vi "RTM CreateFramesChannels.vi"(8 "error in (no error)":errorcluster, 10 "Frame":string="Tx FRAME ", 11 "Node Ptr":T1 format="%.0x") -> (0 "error out":errorcluster, 3 "Node Ptr 2":T1 format="%.0x")   [LabVIEW 2018, in "CAN Gateway System Explorer.lvlib"]
uses:
  CAN Gateway System Explorer.lvlib
  <vilib>/NI Veristand/Custom Device API/Custom Device Item Ref.ctl
  <vilib>/NI Veristand/Custom Device Tools/Custom Device Utility Library/Search Direction.ctl
  <vilib>/NI Veristand/Custom Device API/Custom Device Channel.ctl
  <vilib>/NI Veristand/Custom Device API/Custom Device Channel Type.ctl
  Shared/Constants.vi
  <vilib>/NI Veristand/Custom Device Tools/Custom Device Utility Library/NI VeriStand - Search for Item by GUID.vi
  <vilib>/NI Veristand/Custom Device API/Get Item Property (String).vi
  <vilib>/NI Veristand/Custom Device API/Set Item Property (Boolean).vi
  <resource>/objmgr/xnet.rc
  <vilib>/NI Veristand/Custom Device Tools/Custom Device Utility Library/Custom Device Utility Library.lvlib
  Shared/CAN Gateway Shared.lvlib
  <vilib>/NI Veristand/Custom Device API/Custom Device API.lvlib
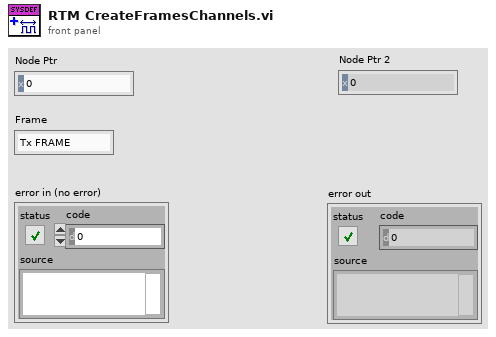
[diagram p1: front panel]
types:
  T1 = typedef "Custom Device API.lvlib/Custom Device Item Ref.ctl" = u64
  T2 = typedef "Custom Device Utility Library.lvlib/Search Direction.ctl" = enum16{"Down", "Up"}
  T3 = typedef "Custom Device API.lvlib/Custom Device Channel.ctl" = cluster{"Type":T4, "Units":string, "Default Value":dbl, "Faultable":bool, "Scalable":bool}
  T4 = typedef "Custom Device API.lvlib/Custom Device Channel Type.ctl" = enum16{"Input", "Output"}
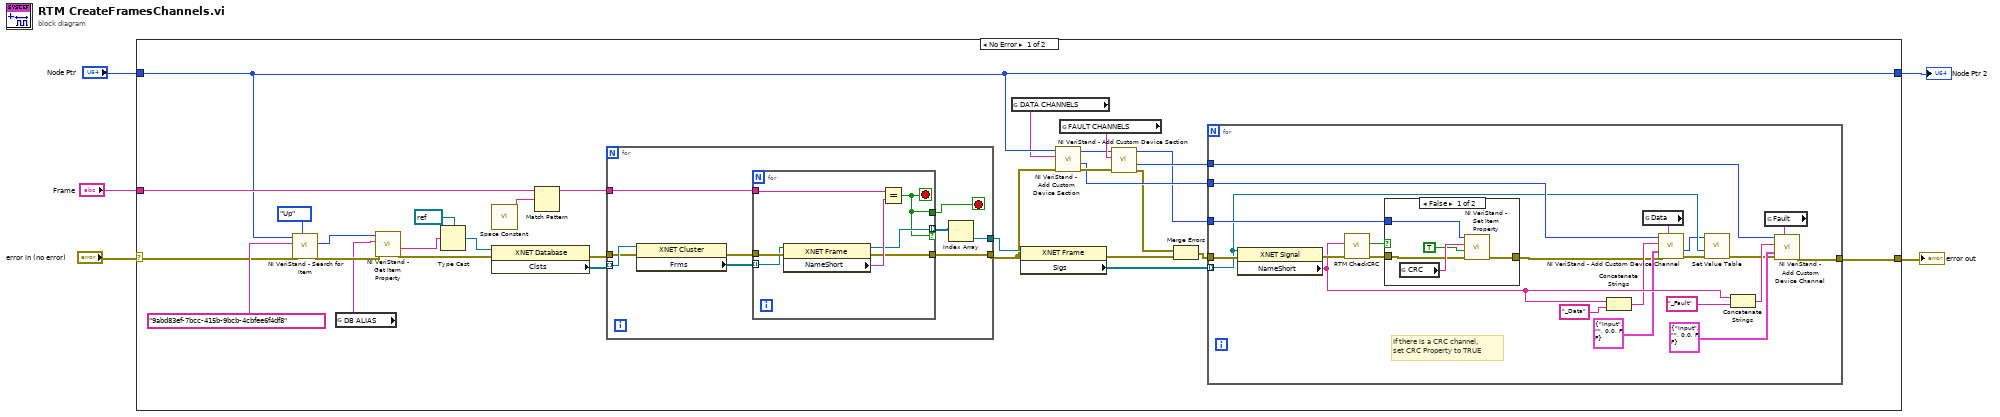
[diagram p0: block diagram]
diagram:
  n1 = case shown="No Error" "error in (no error)" {
    selector: "error in (no error)" -> [w31 w80]
    tunnel: "Node Ptr" -> [w16 w81]
    tunnel: "Frame" -> [w22 _]
    tunnel: [w16 w81] -> w2
    tunnel: [w18 w80] -> w1
    frame No Error {
      n2 = call-poly <vilib>:"NI VeriStand - Search for Item.vi"("Direction (Down)"=Search_Direction."Up", "error in"=w31, "Item GUID"="9abd83ef-7bcc-415b-9bcb-4cbfee6f4df8", "Section Ref in"=w16) -> ("error out"=w34:errorcluster, "Item Ref"=w32:T1)  [unwired: 4 in, 2 out]
      n3 = global read "Constants.vi" "DB ALIAS"() -> (w33:string)
      n4 = call-poly <vilib>:"NI VeriStand - Get Item Property.vi"("error in (no error)"=w34, "Property Name"=w33, "Item Ref in"=w32) -> ("error out"=w28:errorcluster, "Value"=w29:string)  [unwired: 5 in, 2 out]
      n5 = Type Cast(type=refnum<k21> refnum ("XNET Database"), x=w29) -> (*(type *) &x=w27:refnum<k21>)
      n6 = call <vilib>:"Space Constant.vi"() -> ("String"=w21:string)
      n7 = property class="XNET Database"(reference=w27, error in=w28) -> (error out=w25:errorcluster, "Clsts"=w26:refnum<k21>[])  [unwired: 1 out]
      n8 = Match Pattern(string=w22, regular expression=w21) -> (before substring=w20:string)  [unwired: 1 in, 3 out]
      n9 = for {
        tunnel: w26 -> [w72] mode=indexing
        tunnel: w25 -> [w71]
        tunnel: w20 -> [w68]
        tunnel: [w66] -> w24
        tunnel: [w65] -> w17
        stop <- w64 stop-if-true
        n10 = property class="XNET Cluster"(reference=w72, error in=w71) -> (error out=w70:errorcluster, "Frms"=w69:refnum<k21>[])  [unwired: 1 out]
        n11 = for {
          tunnel: w70 -> [w79]
          tunnel: w69 -> [w78] mode=indexing
          tunnel: w68 -> [w77]
          tunnel: [w75] -> w65
          tunnel: [w74] -> w67 mode=indexing if=w73
          tunnel: [w73] -> w64
          stop <- w73 stop-if-true
          n12 = property class="XNET Frame"(reference=w78, error in=w79) -> (reference out=w74:refnum<k21>, error out=w75:errorcluster, "NameShort"=w76:string)
          n13 = Equal?(x=w77, y=w76) -> (x = y?=w73:bool)
        }
        n14 = Index Array(array=w67) -> (element=w66:refnum<k21>)  [unwired: 1 in]
      }
      n15 = global read "Constants.vi" "DATA CHANNELS"() -> (w15:string)
      n16 = property class="XNET Frame"(reference=w24, error in=w17) -> (error out=w7:errorcluster, "Sigs"=w23:refnum<k21>[])  [unwired: 1 out]
      n17 = call <vilib>:"NI VeriStand - Add Custom Device Section.vi"("error in (no error)"=w17, "Section Name"=w15, "Parent Ref in"=w16) -> ("error out"=w13:errorcluster, "Section Ptr"=w11:T1, "Parent Ref out"=w12:T1)  [unwired: 5 in, 1 out]
      n18 = global read "Constants.vi" "FAULT CHANNELS"() -> (w14:string)
      n19 = call <vilib>:"NI VeriStand - Add Custom Device Section.vi"("error in (no error)"=w13, "Section Name"=w14, "Parent Ref in"=w12) -> ("error out"=w6:errorcluster, "Section Ptr"=w10:T1, "Parent Ref out"=w8:T1)  [unwired: 5 in, 1 out]
      n20 = Merge Errors(w6, w7) -> (w9:errorcluster)
      n21 = for {
        tunnel: w23 -> [w37] mode=indexing
        tunnel: w9 -> [w57]
        tunnel: w8 -> [w42]
        tunnel: [w56] -> w18
        tunnel: w11 -> [w41]
        tunnel: w10 -> [w40]
        # "If there is a CRC channel,\nset CRC Property to TRUE"
        n22 = property class="XNET Signal"(reference=w37, error in=w57) -> (error out=w55:errorcluster, "NameShort"=w54:string)  [unwired: 1 out]
        n23 = call "RTM CheckCRC.vi"("error in (no error)"=w55, "SignalName"=w54) -> ("error out"=w45:errorcluster, "CRC?"=w43:bool)  [unwired: 7 in, 1 out]
        n24 = case shown="False" w43 {
          tunnel: w45 -> [w60 w63]
          tunnel: [w59 w63] -> w44
          tunnel: w42 -> [w58 _]
          frame False {
            n25 = global read "Constants.vi" "CRC"() -> (w62:string)
            n26 = call-poly <vilib>:"NI VeriStand - Set Item Property.vi"("error in (no error)"=w60, "Value"=TRUE, "Property Name"=w62, "Item Ref in"=w58) -> ("error out"=w59:errorcluster)  [unwired: 5 in, 2 out]
          }
          frame True {
          }
        }
        n27 = Concatenate Strings(w54, "_Data" ("string")) -> (w50:string)
        n28 = global read "Constants.vi" "Data"() -> (w52:string)
        n29 = call <vilib>:"NI VeriStand - Add Custom Device Channel.vi"("GUID (Default Channel)"=w52, "error in (no error)"=w44, "Channel"=T3 {"Type"=enum."Input", "Units"="", "Default Value"=0.0, "Faultable"=FALSE, "Scalable"=FALSE}, "Channel Name"=w50, "Parent Ref in"=w41) -> ("error out"=w39:errorcluster, "Channel Ref"=w36:T1)  [unwired: 3 in, 2 out]
        n30 = call "Set Value Table.vi"("error in (no error)"=w39, "XNET Signal"=w37, "Channel Ref in"=w36) -> ("error out"=w38:errorcluster)  [unwired: 8 in]
        n31 = Concatenate Strings(w54, "_Fault" ("string")) -> (w48:string)
        n32 = global read "Constants.vi" "Fault"() -> (w46:string)
        n33 = call <vilib>:"NI VeriStand - Add Custom Device Channel.vi"("GUID (Default Channel)"=w46, "error in (no error)"=w38, "Channel"=T3 {"Type"=enum."Input", "Units"="", "Default Value"=0.0, "Faultable"=FALSE, "Scalable"=FALSE}, "Channel Name"=w48, "Parent Ref in"=w40) -> ("error out"=w56:errorcluster)  [unwired: 3 in, 3 out]
      }
    }
    frame Error {
    }
  }
  "error out" <- w1
  "Node Ptr 2" <- w2
